vi "Main.vi"() -> ()   [LabVIEW 2020]
uses:
  Support/Support.lvlib
  Display Console/DisplayConsole.lvlib
  Sensor Interface/SensorInterface.lvlib
  User Console/UserConsole.lvlib
  Error Handler/ErrorHandler.lvlib
  Controller/Controller.lvlib
panel:
  in  "Use Simulated Configuration Database?":bool
  out "error out":errorcluster
  in  "Use Simulated Display Console?":bool
  in  "Use Simulated Display Console?":bool
  in  "Use Simulated Display Console?":bool
  # "[Covers: SI2]"
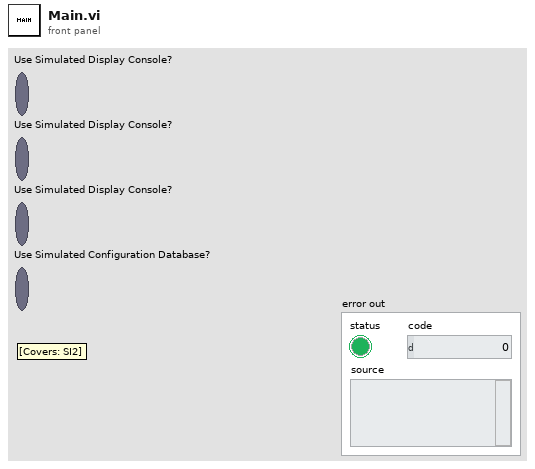
[diagram p1: front panel]
types:
  T1 = typedef "Support.lvlib/Project Messaging Structures.ctl" = cluster{">>EventHandlers":refnum<user-event>, ">>ErrorQ":refnum<queue>, ">>ControllerQ":refnum<queue>}
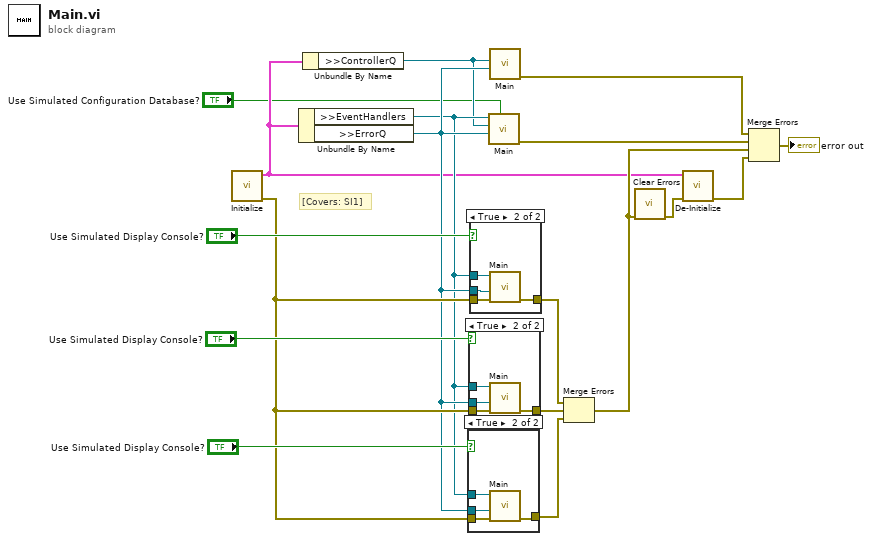
[diagram p0: block diagram]
diagram:
  # "[Covers: SI1]"
  n1 = call "Initialize.vi"() -> ("error out"=w15:errorcluster, "Messaging Structures"=w7:T1)  [unwired: 10 in]
  n2 = Unbundle By Name(w7) -> (">>EventHandlers"=w8:refnum<user-event>, ">>ErrorQ"=w9:refnum<queue>)
  n3 = Unbundle By Name(w7) -> (">>ControllerQ"=w6:refnum<queue>)
  n4 = case shown="True" "Use Simulated Display Console?" {
    tunnel: w15 -> [w19 w23]
    tunnel: [w19 w22] -> w12
    tunnel: w8 -> [_ w21]
    tunnel: w9 -> [_ w20]
    frame False {
    }
    frame True {
      n5 = call "Main.vi"("error in"=w23, ">>ErrorQ"=w20, ">>EventHandlers"=w21) -> ("error out"=w22:errorcluster)  [unwired: 8 in]
    }
  }
  n6 = case shown="True" "Use Simulated Display Console?" {
    tunnel: w15 -> [w24 w28]
    tunnel: [w24 w27] -> w14
    tunnel: w8 -> [_ w26]
    tunnel: w9 -> [_ w25]
    frame False {
    }
    frame True {
      n7 = call "Main.vi"("error in"=w28, ">>ErrorQ"=w25, ">>EventHandlers"=w26) -> ("error out"=w27:errorcluster)  [unwired: 8 in]
    }
  }
  n8 = case shown="True" "Use Simulated Display Console?" {
    tunnel: w15 -> [w29 w33]
    tunnel: [w29 w32] -> w13
    tunnel: w8 -> [_ w31]
    tunnel: w9 -> [_ w30]
    frame False {
    }
    frame True {
      n9 = call "Main.vi"("error in"=w33, ">>ErrorQ"=w30, ">>EventHandlers"=w31) -> ("error out"=w32:errorcluster)  [unwired: 8 in]
    }
  }
  n10 = call "Main.vi"("Is Simulated?"="Use Simulated Configuration Database?", ">>ErrorQ"=w9, ">>ControllerQ"=w6, ">>EventHandlers"=w8) -> ("error out"=w4:errorcluster)  [unwired: 7 in]
  n11 = call "Main.vi"(">>ErrorQ"=w9, ">>ControllerQ"=w6) -> ("error out"=w3:errorcluster)  [unwired: 9 in]
  n12 = Merge Errors(w13, w14, w12) -> (w11:errorcluster)
  n13 = call <vilib>:"Clear Errors.vi"("error in (no error)"=w11) -> ("error out"=w10:errorcluster)  [unwired: 5 in, 1 out]
  n14 = call "De-Initialize.vi"("error in"=w10, "Messaging Structures"=w7) -> ("error out"=w5:errorcluster)  [unwired: 9 in]
  n15 = Merge Errors(w3, w4, w11, w5) -> (→"error out":errorcluster)
